vi "adam5000-chassis-engineering-VI.vi"(0 "VISA Refnum in":refnum<visa-resource-name>, 1 "adam5000:module-type-select":T13, 2 "Chassis Settings in":T14={"VISA resource name"="COM8", "baud rate (19200)"=19200, "Chassis ID"=1}, 5 "adam5000:all-data-in":T3, 7 "adam5000:DO-ch":T12, 9 "adam5000:AO-ch":T11, 11 "error in (no error)":errorcluster, 12 "adam-chassis-cmd-ack":T1, 13 "adam5000:status-ref":T10) -> (4 "VISA Refnum out":refnum<visa-resource-name>, 6 "adam5000:all-data-out":T3, 14 "adam-chassis-cmd-response-out":T1, 15 "error out":errorcluster)   [LabVIEW 2020]
uses:
  controls/thermocouple-input-cluster.ctl
  controls/analog-input-cluster.ctl
  controls/analog-output-cluster.ctl
  controls/digitial-input-cluster.ctl
  controls/digital-output-cluster.ctl
  controls/adam-5000-all-module-datas.ctl
  controls/adam-5000-all-chassis-data.ctl
  controls/adam-5000-serial-settings.ctl
  controls/adam-5000-chassis-module-types.ctl
  controls/adam-5000-AO-user-input.ctl
  controls/adam-5000-cmd-response.ctl
  controls/adam-5000-chassis-cmd-ack.ctl
  controls/adam-5000-status-indicator-references.ctl
  controls/adam-5000-DO-user-input.ctl
panel:
  out "Current Slot":i32
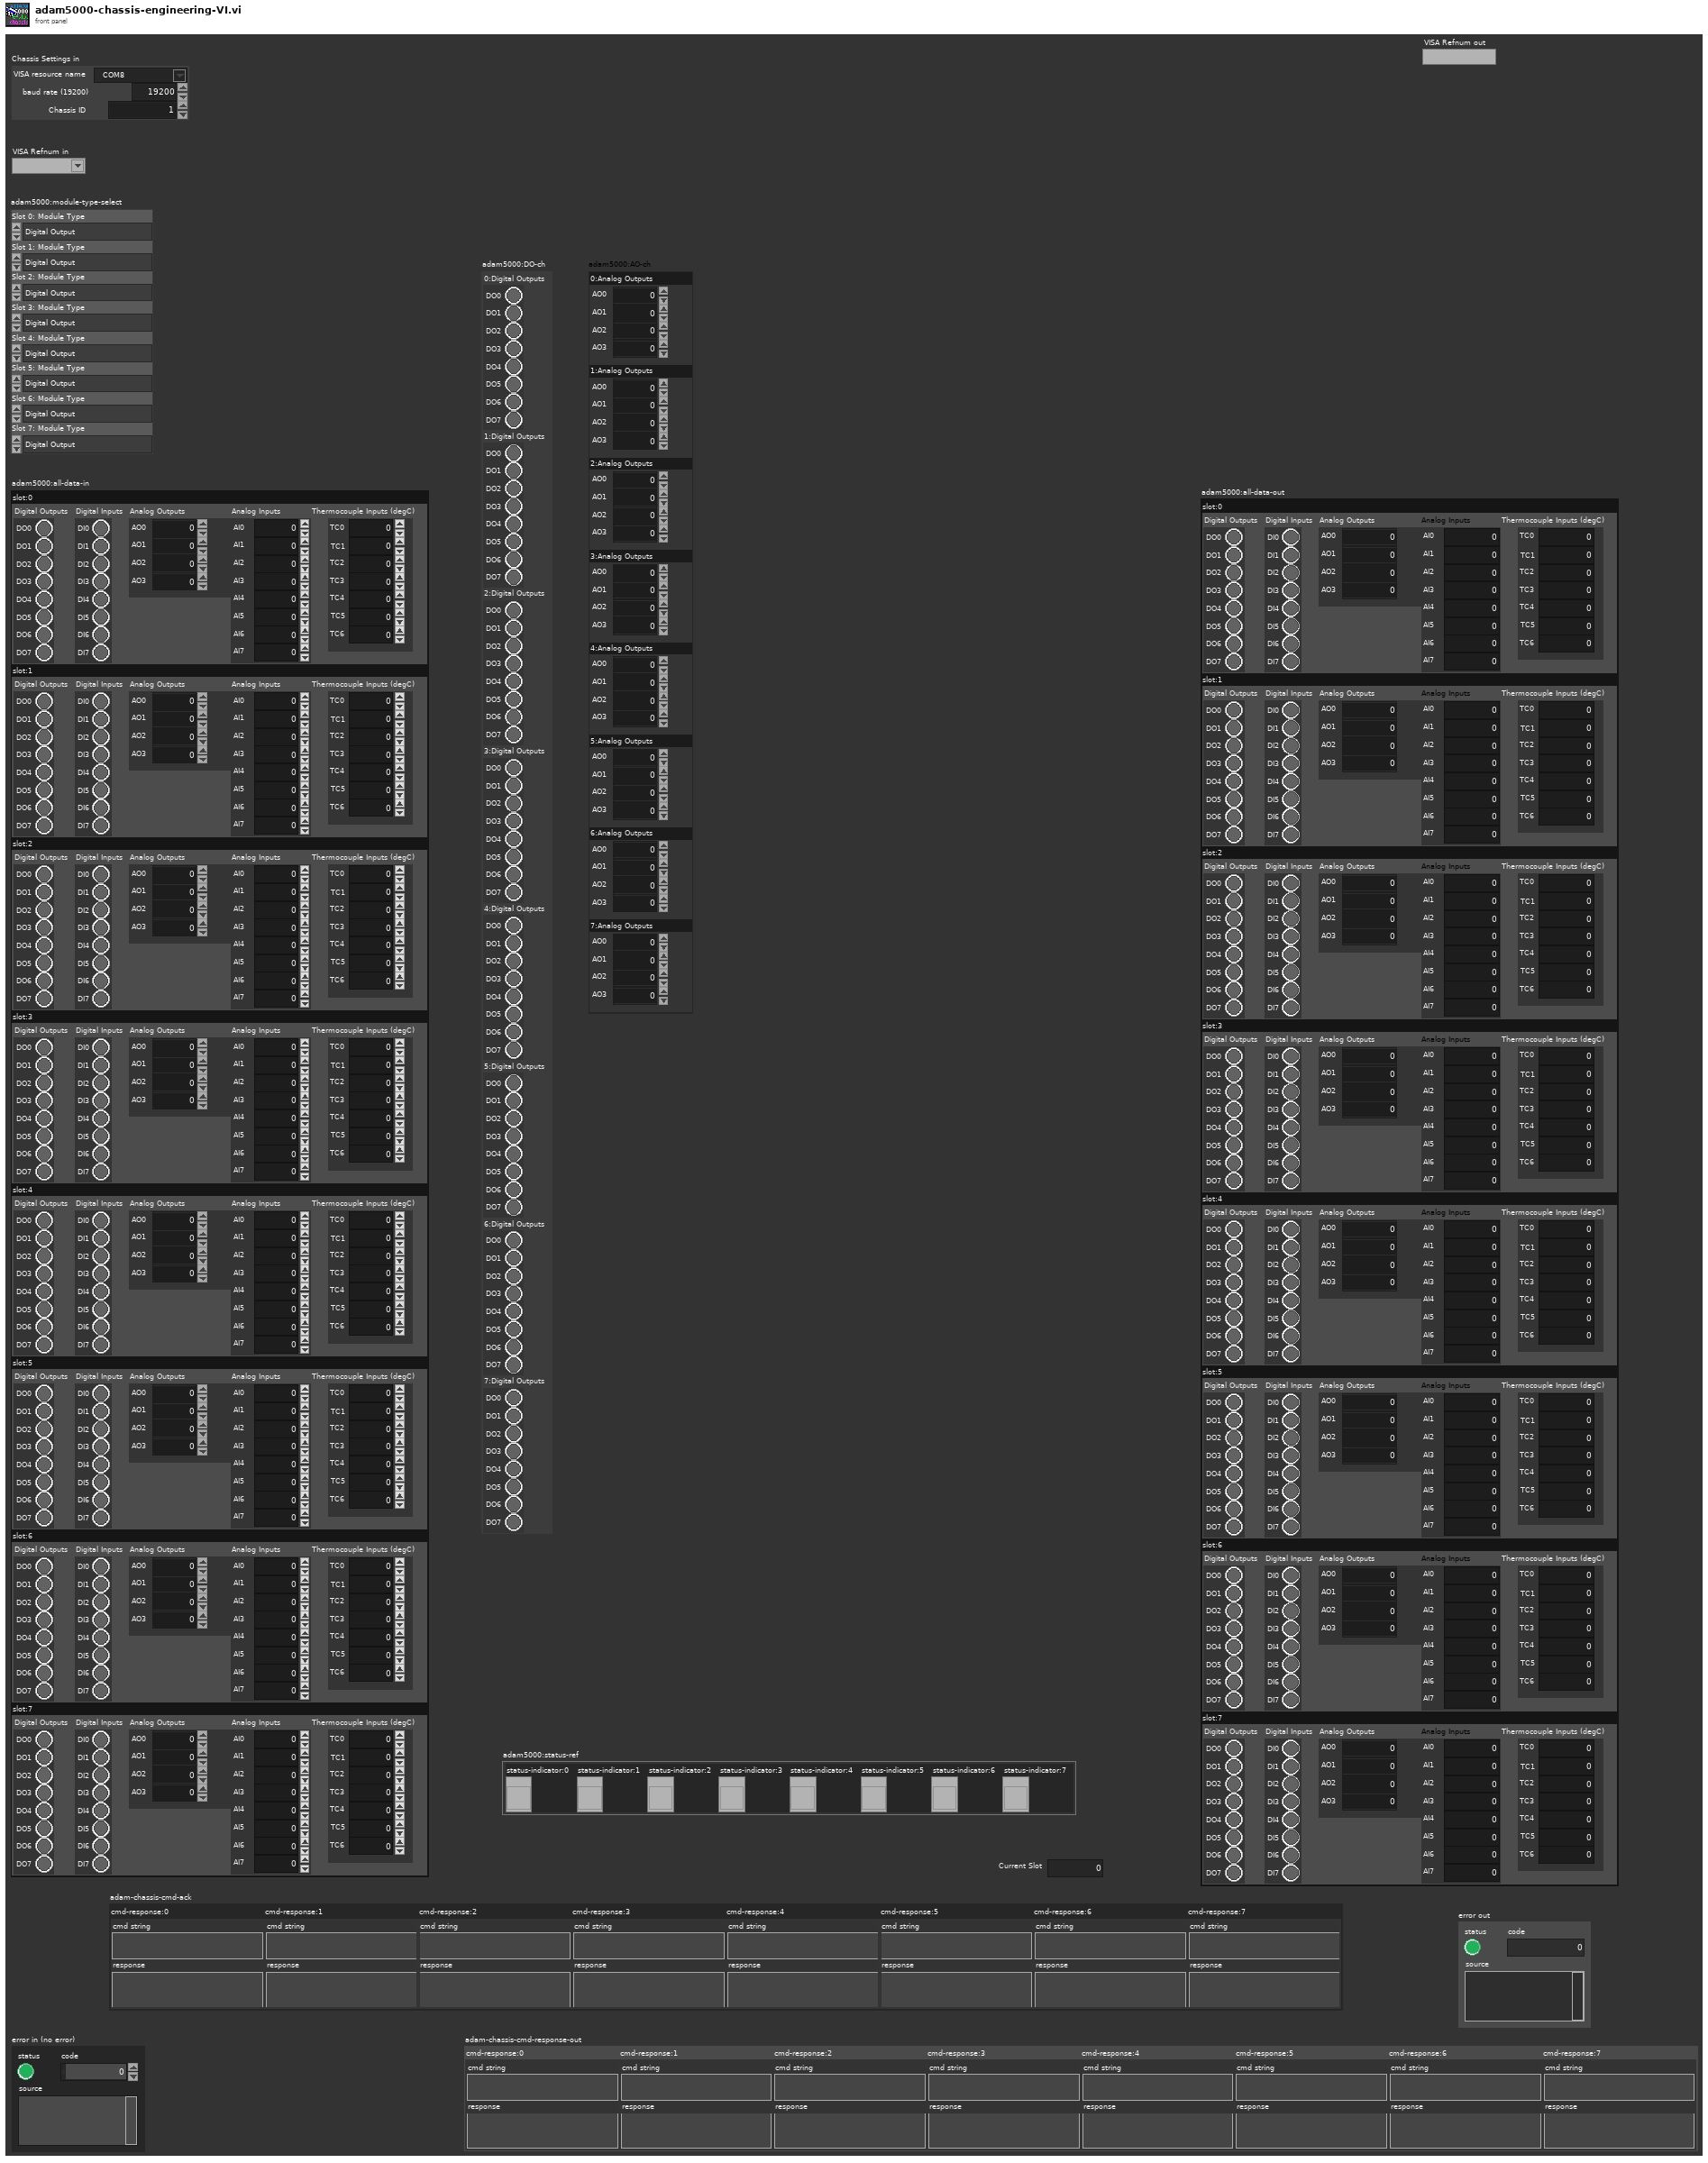
[diagram p1: front panel]
types:
  T1 = typedef "adam-5000-chassis-cmd-ack.ctl" = cluster{"cmd-response:0":T2, "cmd-response:1":T2, "cmd-response:2":T2, "cmd-response:3":T2, "cmd-response:4":T2, "cmd-response:5":T2, "cmd-response:6":T2, "cmd-response:7":T2}
  T2 = typedef "adam-5000-cmd-response.ctl" = cluster{"cmd string":string, "response":string}
  T3 = typedef "adam-5000-all-chassis-data.ctl" = cluster{"slot:0":T4, "slot:1":T4, "slot:2":T4, "slot:3":T4, "slot:4":T4, "slot:5":T4, "slot:6":T4, "slot:7":T4}
  T4 = typedef "adam-5000-all-module-datas.ctl" = cluster{"Digital Outputs":T5, "Digital Inputs":T6, "Analog Outputs":T7, "Analog Inputs":T8, "Thermocouple Inputs (degC)":T9}
  T5 = typedef "digital-output-cluster.ctl" = cluster{"DO0":bool, "DO1":bool, "DO2":bool, "DO3":bool, "DO4":bool, "DO5":bool, "DO6":bool, "DO7":bool}
  T6 = typedef "digitial-input-cluster.ctl" = cluster{"DI0":bool, "DI1":bool, "DI2":bool, "DI3":bool, "DI4":bool, "DI5":bool, "DI6":bool, "DI7":bool}
  T7 = typedef "analog-output-cluster.ctl" = cluster{"AO0":dbl, "AO1":dbl, "AO2":dbl, "AO3":dbl}
  T8 = typedef "analog-input-cluster.ctl" = cluster{"AI0":dbl, "AI1":dbl, "AI2":dbl, "AI3":dbl, "AI4":dbl, "AI5":dbl, "AI6":dbl, "AI7":dbl}
  T9 = typedef "thermocouple-input-cluster.ctl" = cluster{"TC0":dbl, "TC1":dbl, "TC2":dbl, "TC3":dbl, "TC4":dbl, "TC5":dbl, "TC6":dbl}
  T10 = typedef "adam-5000-status-indicator-references.ctl" = cluster{"status-indicator:0":refnum<vi>, "status-indicator:1":refnum<vi>, "status-indicator:2":refnum<vi>, "status-indicator:3":refnum<vi>, "status-indicator:4":refnum<vi>, "status-indicator:5":refnum<vi>, "status-indicator:6":refnum<vi>, "status-indicator:7":refnum<vi>}
  T11 = typedef "adam-5000-AO-user-input.ctl" = cluster{"0:Analog Outputs":T7, "1:Analog Outputs":T7, "2:Analog Outputs":T7, "3:Analog Outputs":T7, "4:Analog Outputs":T7, "5:Analog Outputs":T7, "6:Analog Outputs":T7, "7:Analog Outputs":T7}
  T12 = typedef "adam-5000-DO-user-input.ctl" = cluster{"0:Digital Outputs":T5, "1:Digital Outputs":T5, "2:Digital Outputs":T5, "3:Digital Outputs":T5, "4:Digital Outputs":T5, "5:Digital Outputs":T5, "6:Digital Outputs":T5, "7:Digital Outputs":T5}
  T13 = typedef "adam-5000-chassis-module-types.ctl" = cluster{"Slot 0: Module Type":enum16{"Digital Output", "Digital Input", "Analog Output", "Analog Input", "Thermocouple", "Power Relay", "empty"}, "Slot 1: Module Type":enum16{"Digital Output", "Digital Input", "Analog Output", "Analog Input", "Thermocouple", "Power Relay", "empty"}, "Slot 2: Module Type":enum16{"Digital Output", "Digital Input", "Analog Output", "Analog Input", "Thermocouple", "Power Relay", "empty"}, "Slot 3: Module Type":enum16{"Digital Output", "Digital Input", "Analog Output", "Analog Input", "Thermocouple", "Power Relay", "empty"}, "Slot 4: Module Type":enum16{"Digital Output", "Digital Input", "Analog Output", "Analog Input", "Thermocouple", "Power Relay", "empty"}, "Slot 5: Module Type":enum16{"Digital Output", "Digital Input", "Analog Output", "Analog Input", "Thermocouple", "Power Relay", "empty"}, "Slot 6: Module Type":enum16{"Digital Output", "Digital Input", "Analog Output", "Analog Input", "Thermocouple", "Power Relay", "empty"}, "Slot 7: Module Type":enum16{"Digital Output", "Digital Input", "Analog Output", "Analog Input", "Thermocouple", "Power Relay", "empty"}}
  T14 = typedef "adam-5000-serial-settings.ctl" = cluster{"VISA resource name":refnum<visa-resource-name>, "baud rate (19200)":u32, "Chassis ID":u8}
  T15 = enum16{"Digital Output", "Digital Input", "Analog Output", "Analog Input", "Thermocouple", "Power Relay", "empty"}[]
  T16 = typedef "adam-module-select-tab.ctl" = enum32{"DO", "DI", "AO", "AI", "T/C", ""}
  T17 = cluster{"[0]":T4, "[1]":T4, "[2]":T4, "[3]":T4, "[4]":T4, "[5]":T4, "[6]":T4, "[7]":T4, "[8]":T4}
  T18 = cluster{"[0]":T2, "[1]":T2, "[2]":T2, "[3]":T2, "[4]":T2, "[5]":T2, "[6]":T2, "[7]":T2, "[8]":T2}
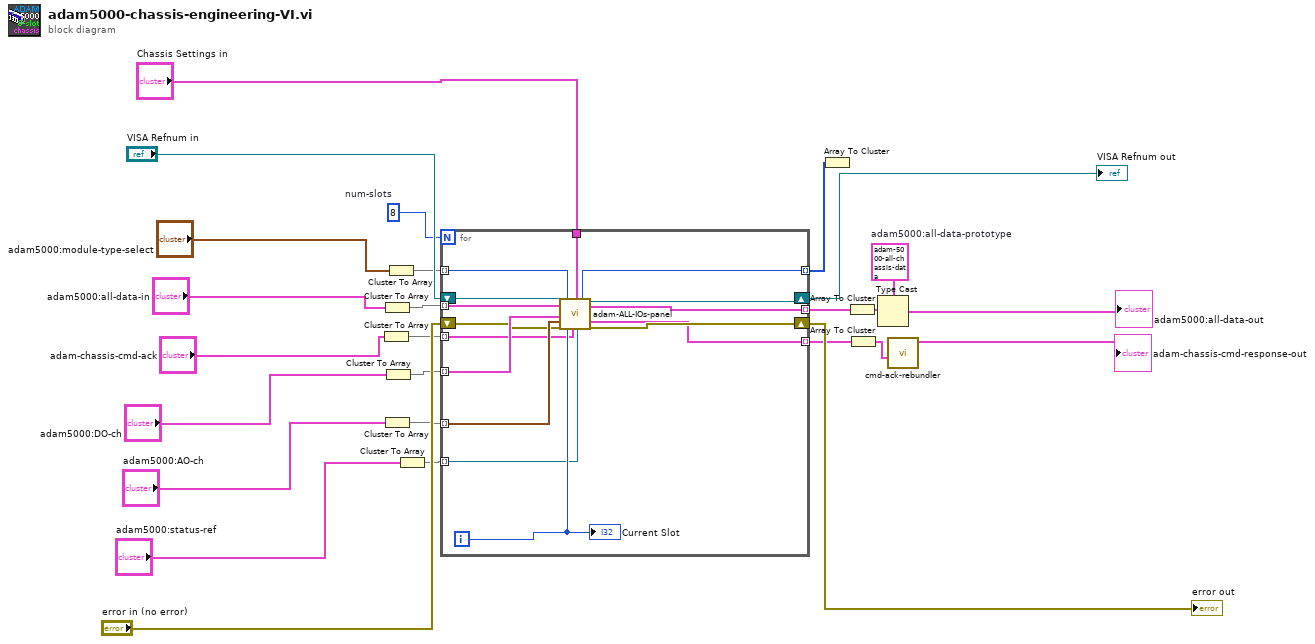
[diagram p0: block diagram]
diagram:
  w9 = T3 {"slot:0"={"Digital Outputs"={"DO0"=FALSE, "DO1"=FALSE, "DO2"=FALSE, "DO3"=FALSE, "DO4"=FALSE, "DO5"=FALSE, "DO6"=FALSE, "DO7"=FALSE}, "Digital Inputs"={"DI0"=FALSE, "DI1"=FALSE, "DI2"=FALSE, "DI3"=FALSE, "DI4"=FALSE, "DI5"=FALSE, "DI6"=FALSE, "DI7"=FALSE}, "Analog Outputs"={"AO0"=0.0, "AO1"=0.0, "AO2"=0.0, "AO3"=0.0}, "Analog Inputs"={"AI0"=0.0, "AI1"=0.0, "AI2"=0.0, "AI3"=0.0, "AI4"=0.0, "AI5"=0.0, "AI6"=0.0, "AI7"=0.0}, "Thermocouple Inputs (degC)"={"TC0"=0.0, "TC1"=0.0, "TC2"=0.0, "TC3"=0.0, "TC4"=0.0, "TC5"=0.0, "TC6"=0.0}}, "slot:1"={"Digital Outputs"={"DO0"=FALSE, "DO1"=FALSE, "DO2"=FALSE, "DO3"=FALSE, "DO4"=FALSE, "DO5"=FALSE, "DO6"=FALSE, "DO7"=FALSE}, "Digital Inputs"={"DI0"=FALSE, "DI1"=FALSE, "DI2"=FALSE, "DI3"=FALSE, "DI4"=FALSE, "DI5"=FALSE, "DI6"=FALSE, "DI7"=FALSE}, "Analog Outputs"={"AO0"=0.0, "AO1"=0.0, "AO2"=0.0, "AO3"=0.0}, "Analog Inputs"={"AI0"=0.0, "AI1"=0.0, "AI2"=0.0, "AI3"=0.0, "AI4"=0.0, "AI5"=0.0, "AI6"=0.0, "AI7"=0.0}, "Thermocouple Inputs (degC)"={"TC0"=0.0, "TC1"=0.0, "TC2"=0.0, "TC3"=0.0, "TC4"=0.0, "TC5"=0.0, "TC6"=0.0}}, "slot:2"={"Digital Outputs"={"DO0"=FALSE, "DO1"=FALSE, "DO2"=FALSE, "DO3"=FALSE, "DO4"=FALSE, "DO5"=FALSE, "DO6"=FALSE, "DO7"=FALSE}, "Digital Inputs"={"DI0"=FALSE, "DI1"=FALSE, "DI2"=FALSE, "DI3"=FALSE, "DI4"=FALSE, "DI5"=FALSE, "DI6"=FALSE, "DI7"=FALSE}, "Analog Outputs"={"AO0"=0.0, "AO1"=0.0, "AO2"=0.0, "AO3"=0.0}, "Analog Inputs"={"AI0"=0.0, "AI1"=0.0, "AI2"=0.0, "AI3"=0.0, "AI4"=0.0, "AI5"=0.0, "AI6"=0.0, "AI7"=0.0}, "Thermocouple Inputs (degC)"={"TC0"=0.0, "TC1"=0.0, "TC2"=0.0, "TC3"=0.0, "TC4"=0.0, "TC5"=0.0, "TC6"=0.0}}, "slot:3"={"Digital Outputs"={"DO0"=FALSE, "DO1"=FALSE, "DO2"=FALSE, "DO3"=FALSE, "DO4"=FALSE, "DO5"=FALSE, "DO6"=FALSE, "DO7"=FALSE}, "Digital Inputs"={"DI0"=FALSE, "DI1"=FALSE, "DI2"=FALSE, "DI3"=FALSE, "DI4"=FALSE, "DI5"=FALSE, "DI6"=FALSE, "DI7"=FALSE}, "Analog Outputs"={"AO0"=0.0, "AO1"=0.0, "AO2"=0.0, "AO3"=0.0}, "Analog Inputs"={"AI0"=0.0, "AI1"=0.0, "AI2"=0.0, "AI3"=0.0, "AI4"=0.0, "AI5"=0.0, "AI6"=0.0, "AI7"=0.0}, "Thermocouple Inputs (degC)"={"TC0"=0.0, "TC1"=0.0, "TC2"=0.0, "TC3"=0.0, "TC4"=0.0, "TC5"=0.0, "TC6"=0.0}}, "slot:4"={"Digital Outputs"={"DO0"=FALSE, "DO1"=FALSE, "DO2"=FALSE, "DO3"=FALSE, "DO4"=FALSE, "DO5"=FALSE, "DO6"=FALSE, "DO7"=FALSE}, "Digital Inputs"={"DI0"=FALSE, "DI1"=FALSE, "DI2"=FALSE, "DI3"=FALSE, "DI4"=FALSE, "DI5"=FALSE, "DI6"=FALSE, "DI7"=FALSE}, "Analog Outputs"={"AO0"=0.0, "AO1"=0.0, "AO2"=0.0, "AO3"=0.0}, "Analog Inputs"={"AI0"=0.0, "AI1"=0.0, "AI2"=0.0, "AI3"=0.0, "AI4"=0.0, "AI5"=0.0, "AI6"=0.0, "AI7"=0.0}, "Thermocouple Inputs (degC)"={"TC0"=0.0, "TC1"=0.0, "TC2"=0.0, "TC3"=0.0, "TC4"=0.0, "TC5"=0.0, "TC6"=0.0}}, "slot:5"={"Digital Outputs"={"DO0"=FALSE, "DO1"=FALSE, "DO2"=FALSE, "DO3"=FALSE, "DO4"=FALSE, "DO5"=FALSE, "DO6"=FALSE, "DO7"=FALSE}, "Digital Inputs"={"DI0"=FALSE, "DI1"=FALSE, "DI2"=FALSE, "DI3"=FALSE, "DI4"=FALSE, "DI5"=FALSE, "DI6"=FALSE, "DI7"=FALSE}, "Analog Outputs"={"AO0"=0.0, "AO1"=0.0, "AO2"=0.0, "AO3"=0.0}, "Analog Inputs"={"AI0"=0.0, "AI1"=0.0, "AI2"=0.0, "AI3"=0.0, "AI4"=0.0, "AI5"=0.0, "AI6"=0.0, "AI7"=0.0}, "Thermocouple Inputs (degC)"={"TC0"=0.0, "TC1"=0.0, "TC2"=0.0, "TC3"=0.0, "TC4"=0.0, "TC5"=0.0, "TC6"=0.0}}, "slot:6"={"Digital Outputs"={"DO0"=FALSE, "DO1"=FALSE, "DO2"=FALSE, "DO3"=FALSE, "DO4"=FALSE, "DO5"=FALSE, "DO6"=FALSE, "DO7"=FALSE}, "Digital Inputs"={"DI0"=FALSE, "DI1"=FALSE, "DI2"=FALSE, "DI3"=FALSE, "DI4"=FALSE, "DI5"=FALSE, "DI6"=FALSE, "DI7"=FALSE}, "Analog Outputs"={"AO0"=0.0, "AO1"=0.0, "AO2"=0.0, "AO3"=0.0}, "Analog Inputs"={"AI0"=0.0, "AI1"=0.0, "AI2"=0.0, "AI3"=0.0, "AI4"=0.0, "AI5"=0.0, "AI6"=0.0, "AI7"=0.0}, "Thermocouple Inputs (degC)"={"TC0"=0.0, "TC1"=0.0, "TC2"=0.0, "TC3"=0.0, "TC4"=0.0, "TC5"=0.0, "TC6"=0.0}}, "slot:7"={"Digital Outputs"={"DO0"=FALSE, "DO1"=FALSE, "DO2"=FALSE, "DO3"=FALSE, "DO4"=FALSE, "DO5"=FALSE, "DO6"=FALSE, "DO7"=FALSE}, "Digital Inputs"={"DI0"=FALSE, "DI1"=FALSE, "DI2"=FALSE, "DI3"=FALSE, "DI4"=FALSE, "DI5"=FALSE, "DI6"=FALSE, "DI7"=FALSE}, "Analog Outputs"={"AO0"=0.0, "AO1"=0.0, "AO2"=0.0, "AO3"=0.0}, "Analog Inputs"={"AI0"=0.0, "AI1"=0.0, "AI2"=0.0, "AI3"=0.0, "AI4"=0.0, "AI5"=0.0, "AI6"=0.0, "AI7"=0.0}, "Thermocouple Inputs (degC)"={"TC0"=0.0, "TC1"=0.0, "TC2"=0.0, "TC3"=0.0, "TC4"=0.0, "TC5"=0.0, "TC6"=0.0}}}  # adam5000:all-data-prototype
  w1 = 8  # num-slots
  n1 = Cluster To Array(cluster="adam-chassis-cmd-ack") -> (array=w4:T2[])
  n2 = Cluster To Array(cluster="adam5000:all-data-in") -> (array=w3:T4[])
  n3 = Cluster To Array(cluster="adam5000:AO-ch") -> (array=w6:T7[])
  n4 = Cluster To Array(cluster="adam5000:DO-ch") -> (array=w5:T5[])
  n5 = Cluster To Array(cluster="adam5000:module-type-select") -> (array=w11:T15)
  n6 = Cluster To Array(cluster="adam5000:status-ref") -> (array=w12:refnum<vi>[])
  n7 = for {
    N: w1 -> [_]
    shift-right: [w32] -> w26
    shift-left: "error in (no error)" -> [w33]
    shift-right: [w38] -> w2
    shift-left: "VISA Refnum in" -> [w37]
    tunnel: w3 -> [w36] mode=indexing
    tunnel: w4 -> [w28] mode=indexing
    tunnel: w5 -> [w35] mode=indexing
    tunnel: w6 -> [w34] mode=indexing
    tunnel: "Chassis Settings in" -> [w40]
    tunnel: w11 -> [w41] mode=indexing
    tunnel: w12 -> [w27] mode=indexing
    tunnel: [w39] -> w13 mode=indexing
    tunnel: [w31] -> w14 mode=indexing
    tunnel: [w30] -> w15 mode=indexing
    i -> [w29]
    n8 = call "adam-ALL-IOs-panel.vi"("VISA Refnum in"=w37, "ADAM-5000-data-current"=w36, "Digital Outputs"=w35, "Analog Outputs"=w34, "error in (no error)"=w33, "Module Type"=w41, "chassis-slot"=w29, "cmd-response in"=w28, "Chassis Settings"=w40, "reference"=w27) -> ("slot: x"=w39:T16, "VISA Refnum out"=w38:refnum<visa-resource-name>, "ADAM-5000-data-new"=w31:T4, "cmd-response out"=w30:T2, "error out"=w32:errorcluster)  [unwired: 5 in]
    "Current Slot" <- w29
  }
  "VISA Refnum out" <- w2
  "error out" <- w26
  n9 = Array To Cluster(array=w13) -> ()  [unwired: 1 out]
  n10 = Array To Cluster(array=w14) -> (cluster=w8:T17)
  n11 = Array To Cluster(array=w15) -> (cluster=w17:T18)
  n12 = Type Cast(type=w9, x=w8) -> (*(type *) &x=→"adam5000:all-data-out":T3)
  n13 = call "cmd-ack-rebundler.vi"("cmd-response-in"=w17) -> ("adam-chassis-cmd-response-out"=→"adam-chassis-cmd-response-out":T1)  [unwired: 10 in]
